vi "Disconnect status checking.vi"(9 "flag":i32[](array[numeric])) -> (2 "failure_flag 1":bool)   [LabVIEW 2016]
uses:
  Communication/Global communication.vi
  Model Management/Global_MdlMgmt.vi
  <vilib>/imath/engines/lvmath2/RunTimeEngine/Managers/WorkSpace/UID Generator.vi
  <vilib>/imath/engines/lvmath2/RunTimeEngine/BuiltInFunctions/size/NIMS_[I32,I32]=size(GRow).vi
  <instcachedir>/0/NIMS_[I32,I32]=size(GRow)_CFE2C4BDC5BC45CD88F2F6A295A2273D.lvgen/NIMS_[I32,I32]=size(GRow)_CFE2C4BDC5BC45CD88F2F6A295A2273D_001.vi
  <vilib>/imath/engines/lvmath2/RunTimeEngine/RangeToken/NIMS_Range_R2 - Integer.vi
  <instcachedir>/0/NIMS_Range_R2 - Integer_89B873E74E6E489885E44F751DD9C6BF.lvgen/NIMS_Range_R2 - Integer_89B873E74E6E489885E44F751DD9C6BF_000.vi
  <vilib>/imath/engines/lvmath2/RunTimeEngine/CommandStatement/MC_CommandStatement_break.vi
  <vilib>/imath/engines/lvmath2/RunTimeEngine/IndexRead/NIMS M($,S).vi
  <instcachedir>/0/NIMS M($,S)_3E5749BBB62E49528D4765A77F1F6D98.lvgen/NIMS M($,S)_3E5749BBB62E49528D4765A77F1F6D98_000.vi
  <vilib>/imath/engines/lvmath2/RunTimeEngine/BuiltInFunctions/findnz/NIMS_[3o]_findnz(GColV).vi
  <instcachedir>/0/NIMS_[3o]_findnz(GColV)_E56CE4C0B89545728115E0FFBA09CCA4.lvgen/NIMS_[3o]_findnz(GColV)_E56CE4C0B89545728115E0FFBA09CCA4_000.vi
  <vilib>/imathl/engines/lvmath/Functions/Error Handling/Create Error.vi
  <vilib>/imath/engines/lvmath2/RunTimeEngine/BuiltInFunctions/is_empty/NIMS_is_empty(GV).vi
  <instcachedir>/0/NIMS_is_empty(GV)_FC7E7C3D9544432CB6AA2416ADCF6D56.lvgen/NIMS_is_empty(GV)_FC7E7C3D9544432CB6AA2416ADCF6D56_000.vi
  <vilib>/imath/engines/lvmath2/RunTimeEngine/BuiltInFunctions/size/NIMS_[I32,I32]=size(GCol).vi
  <instcachedir>/0/NIMS_[I32,I32]=size(GCol)_E415432306A64FB2A9F0B693E1D4163C.lvgen/NIMS_[I32,I32]=size(GCol)_E415432306A64FB2A9F0B693E1D4163C_000.vi
  <vilib>/imath/engines/lvmath2/RunTimeEngine/IndexRead/NIMS V(S).vi
  <instcachedir>/0/NIMS V(S)_0488751826AF41519A22953C041130DC.lvgen/NIMS V(S)_0488751826AF41519A22953C041130DC_002.vi
  <instcachedir>/0/NIMS V(S)_0488751826AF41519A22953C041130DC.lvgen/NIMS V(S)_0488751826AF41519A22953C041130DC_000.vi
  <vilib>/imath/engines/lvmath2/RunTimeEngine/ErrorHandling/NIMS_Create Error From Enums.vi
  <vilib>/imath/engines/lvmath2/RunTimeEngine/RunTimeType/NIMS_RunTimeType_From StrictType (excl LVString).vi
  <instcachedir>/0/NIMS_RunTimeType_From StrictType (excl LVString)_BBF44FB49F834B71AF7A14CCEDF8BECD.lvgen/NIMS_RunTimeType_From StrictType (excl LVString)_BBF44FB49F834B71AF7A14CCEDF8BECD_000.vi
  <vilib>/imath/engines/lvmath2/RunTimeEngine/LocalVariableDefStatement/MC_LocalVariableDefStatement_Display.vi
  <vilib>/imath/engines/lvmath2/RunTimeEngine/Managers/SymbolTable/Clear UID.vi
  <vilib>/imath/engines/lvmath2/RunTimeEngine/NodeEndStatement/NIMS_NodeEndStatement_Output.vi
  <instcachedir>/0/NIMS_NodeEndStatement_Output_53EC0D466D134D7ABD903AC30B43404B.lvgen/NIMS_NodeEndStatement_Output_53EC0D466D134D7ABD903AC30B43404B_011.vi
  <vilib>/imath/engines/lvmath2/RunTimeEngine/ErrorHandling/NIMS_Finalize Error.vi
  <vilib>/imath/engines/lvmath2/RunTimeEngine/Managers/SymbolTable/NIMS_WorkSpace.lvlib
panel:
  out "x = y?":bool
  in  "=1?":bool
  in  "i>=20?":bool
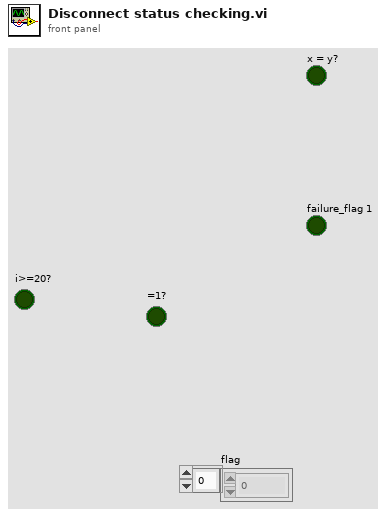
[diagram p1: front panel]
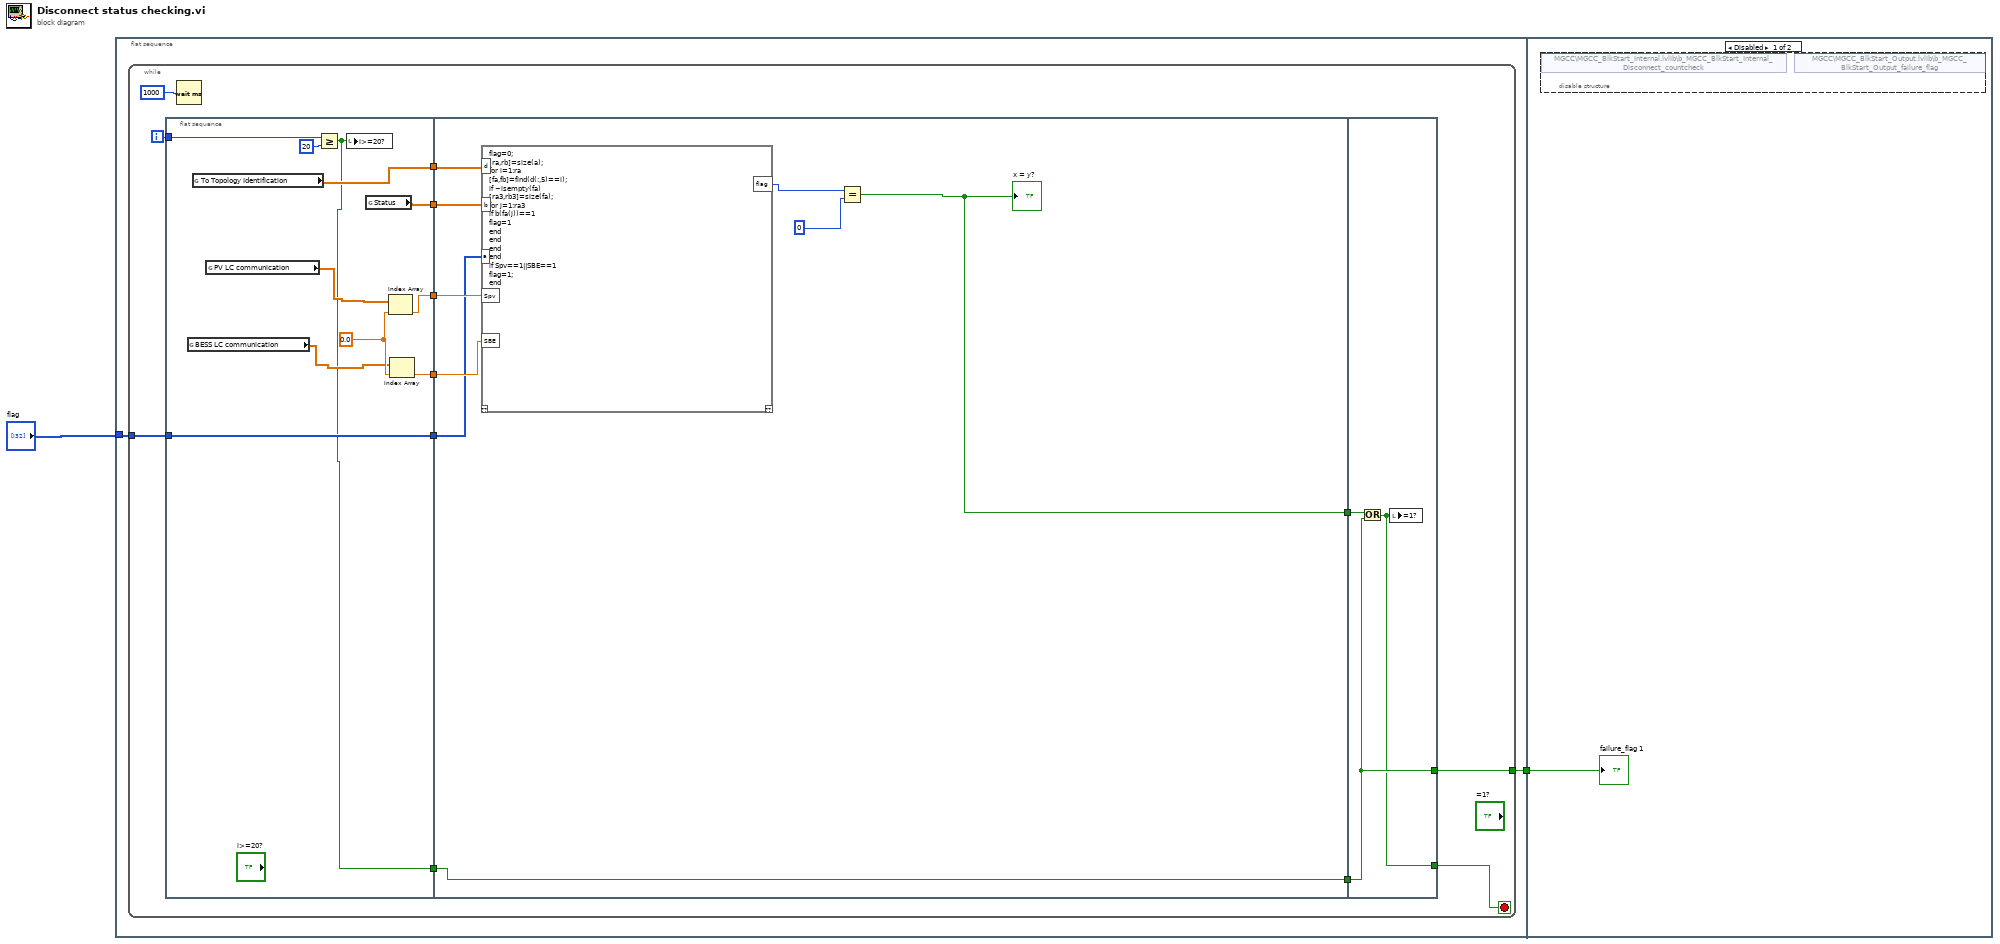
[diagram p0: block diagram]
diagram:
  n1 = flat-sequence {
    tunnel: "flag" -> [w4]
    tunnel: [w3] -> w1
    tunnel: w1 -> [w321]
    frame #0 {
      n2 = while {
        tunnel: w4 -> [w13]
        tunnel: [w11] -> w3
        i -> [w16]
        stop <- w5 stop-if-true
        n3 = flat-sequence {
          tunnel: w16 -> [w28]
          tunnel: w13 -> [w25]
          tunnel: [w25] -> w12
          tunnel: [w26] -> w10
          tunnel: [w21] -> w9
          tunnel: [w23] -> w8
          tunnel: [w22] -> w7
          tunnel: [w18] -> w6
          tunnel: [w37] -> w15
          tunnel: [w29] -> w14
          tunnel: w12 -> [w30]
          tunnel: w10 -> [w36]
          tunnel: w9 -> [w31]
          tunnel: w8 -> [w35]
          tunnel: w7 -> [w34]
          tunnel: w6 -> [w37]
          tunnel: w15 -> [w319]
          tunnel: w14 -> [w320]
          tunnel: [w319] -> w11
          tunnel: [w318] -> w5
          frame #0 {
            w24 = 0.0
            n4 = global read "Global communication.vi" "BESS LC communication"() -> (w19:dbl[])
            n5 = global read "Global_MdlMgmt.vi" "To Topology Identification"() -> (w21:dbl[][])
            n6 = global read "Global communication.vi" "PV LC communication"() -> (w20:dbl[])
            n7 = Greater Or Equal?(x=w28, y=20) -> (x >= y?=w18:bool)
            n8 = local write "i>=20?"(w18) -> ()
            n9 = global read "Global communication.vi" "Status"() -> (w26:dbl[])
            n10 = Index Array(array=w20, index=w24) -> (element=w22:dbl)
            n11 = Index Array(array=w19, index=w24) -> (element=w23:dbl)
          }
          frame #1 {
            n12 = mathscript code="flag=0;\n[ra,rb]=size(a);\nfor i=1:ra\n[fa,fb]=find(d(:,5)==i);\nif ~isempty(fa)\n[ra3,rb3]=size(fa);\nfor j=1:ra3\nif b(fa(j))==1\nflag=1\nend\nend\nend\nend\nif Spv==1||SBE==1\nflag=1;\nend"("d"=w31, "b"=w36, "Spv"=w34, "SBE"=w35, "a"=w30) -> ("flag"=w33:i32)  [unwired: 1 in, 1 out]
            n13 = Equal?(x=w33, y=0) -> (x = y?=w29:bool)
            "x = y?" <- w29
          }
          frame #2 {
            n14 = Or(x=w320, y=w319) -> (x .or. y?=w318:bool)
            n15 = local write "=1?"(w318) -> ()
          }
        }
        n16 = Wait (ms)(milliseconds to wait=1000) -> ()  [unwired: 1 out]
      }
    }
    frame #1 {
      n17 = disable-structure shown="Disabled" {
        frame Disabled {
          n18 = shared-variable "MGCC\\MGCC_BlkStart_Internal.lvlib\\b_MGCC_BlkStart_Internal_Disconnect_countcheck"() -> ()  [unwired: 1 in, 2 out]
          n19 = shared-variable "MGCC\\MGCC_BlkStart_Output.lvlib\\b_MGCC_BlkStart_Output_failure_flag"() -> ()  [unwired: 2 in, 1 out]
        }
        frame Enabled {
        }
      }
      "failure_flag 1" <- w321
    }
  }
